vi "Configure Waveform.vi"(7 "Trace (0: U1)":i32(ring) items=["U1", "I1", "U2", "I2", "U3", "I3", "U4", "I4", "U5", "I5", "U6", "I6", "Speed", "Torque", "AUX1", "AUX2"], 8 "error in (no error)":errorcluster, 9 "End Point (1600)":i32=1600 min=0 max=1601 step=1, 10 "Start Point (0)":i32 min=0 max=1601 step=1, 11 "VISA resource name":refnum<visa-resource-name>) -> (0 "error out":errorcluster, 3 "VISA resource name out":refnum<visa-resource-name>)   [LabVIEW 2021, in "Yokogawa WT1800 Series.lvlib"]
doc: "Configures the waveform features."
uses:
  <instrlib>/Yokogawa WT1800 Series/Yokogawa WT1800 Series.lvlib
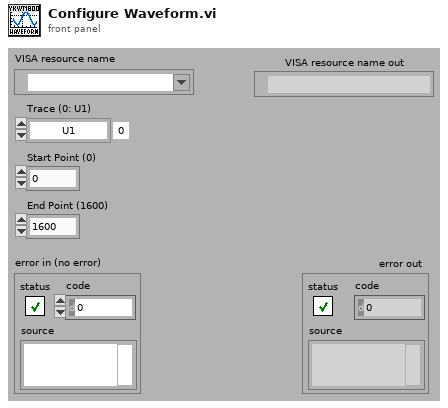
[diagram p1: front panel]
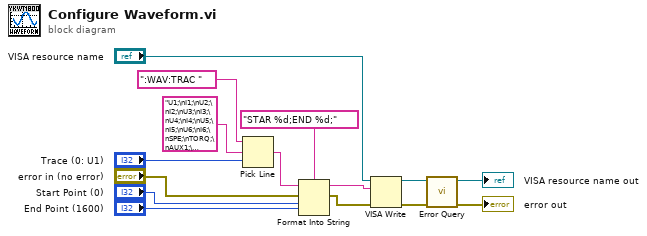
[diagram p0: block diagram]
diagram:
  n1 = Pick Line ("ライン選択")(string ("")=":WAV:TRAC " ("形式文字列"), multi-line string="U1;\nI1;\nU2;\nI2;\nU3;\nI3;\nU4;\nI4;\nU5;\nI5;\nU6;\nI6;\nSPE;\nTORQ;\nAUX1;\nAUX2;" ("複数行文字列"), line index="Trace (0: U1)") -> (output string=w6:string)
  n2 = Format Into String(format string="STAR %d;END %d;" ("形式文字列"), initial string=w6, error in="error in (no error)", "Start Point (0)", "End Point (1600)") -> (resulting string=w2:string, error out=w1:errorcluster)
  n3 = VISA Write ("VISA書き込み")(VISA resource name="VISA resource name", write buffer=w2, error in (no error)=w1) -> (VISA resource name out=w15:refnum<visa-resource-name>, error out=w14:errorcluster)  [unwired: 1 out]
  n4 = call <instrlib>:"Error Query.vi"("error in (no error)"=w14, "VISA resource name"=w15) -> ("error out"=→"error out":errorcluster, "VISA resource name out"=→"VISA resource name out":refnum<visa-resource-name>)  [unwired: 6 in, 2 out]
